vi "Mcp2210 Set Usb Key Params.vi"(8 "error in (no error)":errorcluster, 10 "USB Setting":T1 {"PID" format="%x"; "VID" format="%x"}, 11 "handle":i32) -> (0 "error out":errorcluster, 3 "handle out":i32)   [LabVIEW 2015, in "mcp2210.lvlib"]
doc: "Configures the USB key attributes: VID, PID and power settings.\nIn case of successful execution, the function returns 0 (M_E_SUCCESS).\nIn case of failure, negative error code is returned.\nIf the error code is \"M_E_ERR_BLOCKED_ACCESS\" the write failure is due to the device being either\npassword protected or permanently locked. M_Mcp2210_GetAccessStatus() API provides the details about\ndevice protection status. If the device is not permanently locked, the password protection can be\nunlocked or disabled by using the access control API.\nParameters:\nInputs:\n- IntPtr handle - USB device handle. Cannot be NULL.\n- unsigned short vid - device VID\n- unsigned short pid - device PID\n- unsigned char pwrSrc - device power source, according to USB 2.0 specs, chapter 9:\n- bit 7 = Host-Powered: 1=yes.\nThis bit is reserved and must be set to 1 for historical\nreasons.\n- bit 6 = Self-Powered: 1=yes; 0=no.\n- bits 5..0 must be set to 0 (as an extra safety measure)\n- unsigned char rmtWkup - device is remote wake-up capable: 1=yes; 0=no.\n- unsigned short currentLd - Maximum current consumption from the USB Host, expressed in mA.\nThe value must be a multiple of 2 value, ranging from 2mA to 510mA.\nIf the currentLd value is not multiple by 2, the API will\nround it up to the next multiple by 2 number and store it in NVRAM.\nOutputs:\n- none\nReturns:\n- 0 for success: M_E_SUCCESS\n- negative error code: M_E_ERR_NULL, M_E_ERR_INVALID_HANDLE_VALUE, M_E_ERR_INVALID_PARAMETER\nM_E_ERR_HID_TIMEOUT, M_E_ERR_HID_RW_FILEIO, M_E_ERR_UNKOWN_ERROR\nM_E_ERR_CMD_ECHO, M_E_ERR_CMD_FAILED\nM_E_ERR_BLOCKED_ACCESS\n\nMCP2210_DLL_UM_API int __stdcall Mcp2210_SetUsbKeyParams(void *handle, unsigned short vid, unsigned short pid,\n unsigned char pwrSrc, unsigned char rmtWkup, unsigned short currentLd);"
uses:
  <userlib>/mcp2210/mcp2210.lvlib
  <userlib>/mcp2210/mcp2210_dll_um_x86.dll
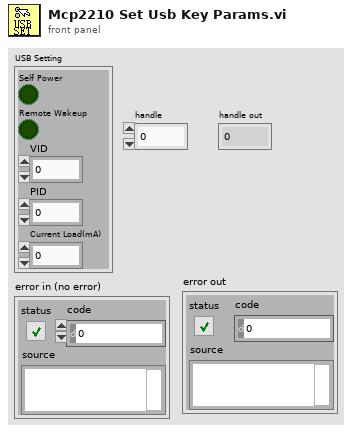
[diagram p1: front panel]
types:
  T1 = cluster{"Self Power":bool, "Remote Wakeup":bool, "VID":u16, "PID":u16, "Current Load(mA)":u16}
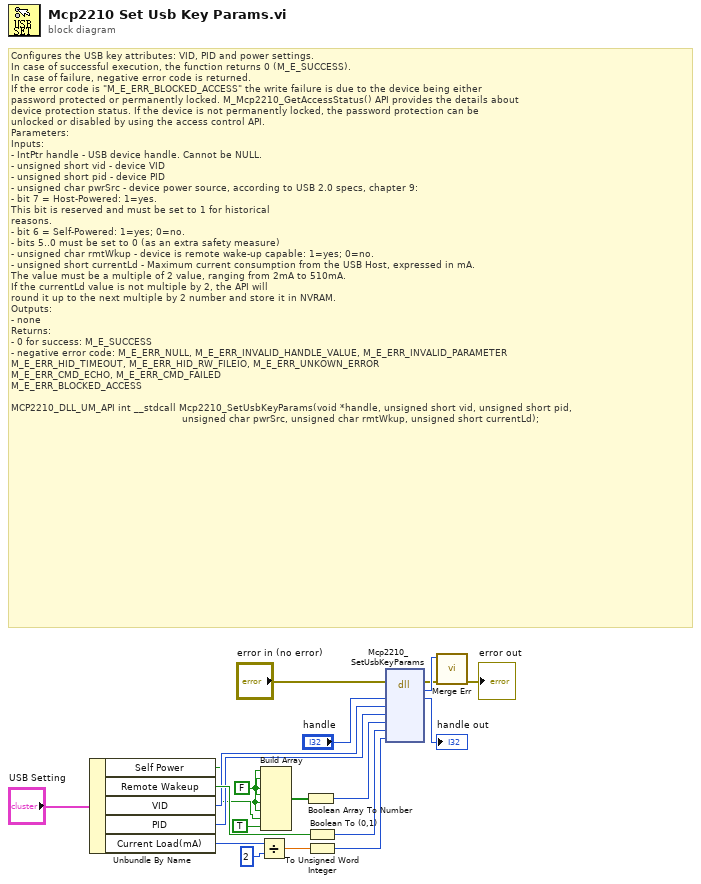
[diagram p0: block diagram]
diagram:
  w1 = FALSE
  # "Configures the USB key attributes: VID, PID and power settings.\nIn case of successful execution, the function returns 0 (M_E_SUCCESS).\nIn case of failure, negative error code is returned.\nIf the error code is \"M_E_ERR_BLOCKED_ACCESS\" the write failure is due to the device being either\npassword protected or permanently locked. M_Mcp2210_GetAccessStatus() API provides the details about\ndevice protection status. If the device is not permanently locked, the password protection can be\nunlocked or disabled by using the access control API.\nParameters:\nInputs:\n- IntPtr handle - USB device handle. Cannot be NULL.\n- unsigned short vid - device VID\n- unsigned short pid - device PID\n- unsigned char pwrSrc - device power source, according to USB 2.0 specs, chapter 9:\n- bit 7 = Host-Powered: 1=yes.\nThis bit is reserved and must be set to 1 for historical\nreasons.\n- bit 6 = Self-Powered: 1=yes; 0=no.\n- bits 5..0 must be set to 0 (as an extra safety measure)\n- unsigned char rmtWkup - device is remote wake-up capable: 1=yes; 0=no.\n- unsigned short currentLd - Maximum current consumption from the USB Host, expressed in mA.\nThe value must be a multiple of 2 value, ranging from 2mA to 510mA.\nIf the currentLd value is not multiple by 2, the API will\nround it up to the next multiple by 2 number and store it in NVRAM.\nOutputs:\n- none\nReturns:\n- 0 for success: M_E_SUCCESS\n- negative error code: M_E_ERR_NULL, M_E_ERR_INVALID_HANDLE_VALUE, M_E_ERR_INVALID_PARAMETER\nM_E_ERR_HID_TIMEOUT, M_E_ERR_HID_RW_FILEIO, M_E_ERR_UNKOWN_ERROR\nM_E_ERR_CMD_ECHO, M_E_ERR_CMD_FAILED\nM_E_ERR_BLOCKED_ACCESS\n\nMCP2210_DLL_UM_API int __stdcall Mcp2210_SetUsbKeyParams(void *handle, unsigned short vid, unsigned short pid,\n                                                         unsigned char pwrSrc, unsigned char rmtWkup, unsigned short currentLd);"
  n1 = Unbundle By Name("USB Setting") -> ("Self Power"=w2:bool, "Remote Wakeup"=w7:bool, "VID"=w6:u16, "PID"=w5:u16, "Current Load(mA)"=w4:u16)
  n2 = Divide(x=w4, y=u16 2) -> (x/y=w17:dbl)
  n3 = Build Array(w1, w1, w1, w1, w1, w1, w2, TRUE ("element")) -> (w14:bool[])
  n4 = Boolean Array To Number(Boolean array=w14) -> (number=w13:u32)
  n5 = Boolean To (0,1)(Boolean=w7) -> (0, 1=w15:i16)
  n6 = To Unsigned Word Integer(number=w17) -> (unsigned 16bit integer=w16:u16)
  n7 = dll-call lib="D:/LabVIEW 2015/user.lib/mcp2210/mcp2210_dll_um_x86.*" fn="Mcp2210_SetUsbKeyParams"(error in="error in (no error)", "handle"="handle", "vid"=w6, "pid"=w5, "pwrSrc"=w13, "rmtWkup"=w15, "currentLd"=w16) -> (error out=w11:errorcluster, "return type"=w12:i32, "handle"=→"handle out":i32)  [unwired: 7 in, 1 out]
  n8 = call <userlib>:"Merge Err.vi"("error in (no error)"=w11, "return type"=w12) -> ("error out"=→"error out":errorcluster)  [unwired: 9 in]
